vi "Send Time-delayed Transfer Sample.vi"(8 "error in (no error)":errorcluster, 9 "Milliseconds To Wait (1000)":i32=1000, 11 "cRIO-CO2 in":refnum<class "cRIO-CO2.lvclass">) -> (0 "error out":errorcluster, 3 "cRIO-CO2 out":refnum<class "cRIO-CO2.lvclass">)   [LabVIEW 2015, in "cRIO-Carbondioxide.lvlib" / "cRIO-CO2.lvlib" / "cRIO-CO2.lvclass"]
uses:
  cRIO-CO2.lvclass
  cRIO-CO2 Messages/Transfer Sample Msg/Transfer Sample Msg.lvclass
  <vilib>/ActorFramework/Time-Delayed Send Message/Time-Delay Override Options.ctl
  <vilib>/ActorFramework/Message/Message.lvclass
  cRIO-CO2.lvclass/cRIO-CO2.ctl
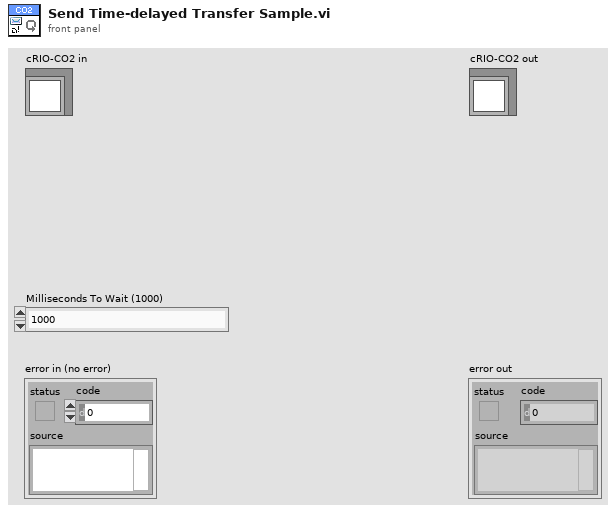
[diagram p1: front panel]
types:
  T1 = typedef "Time-Delay Override Options.ctl" = enum16{"Send next copy now", "Skip next scheduled copy", "Send next copy now and stop all further copies", "Stop all further copies"}
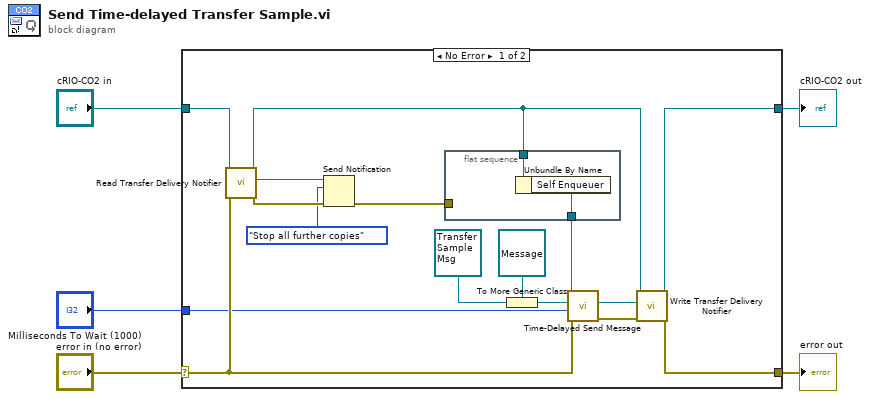
[diagram p0: block diagram]
diagram:
  n1 = case shown="No Error" "error in (no error)" {
    selector: "error in (no error)" -> [w16 w25]
    tunnel: [w17 w25] -> w4
    tunnel: [w18 w24] -> w2
    tunnel: "cRIO-CO2 in" -> [w15 w24]
    tunnel: "Milliseconds To Wait (1000)" -> [w10 _]
    frame No Error {
      n2 = call "Read Transfer Delivery Notifier.vi"("error in (no error)"=w16, "cRIO-CO2 in"=w15) -> ("error out"=w12:errorcluster, "Transfer Delivery Notifier"=w13:refnum<notifier>, "cRIO-CO2 out"=w14:refnum<class "cRIO-CO2.lvclass">)  [unwired: 7 in]
      n3 = Send Notification(notification=Time-Delay_Override_Options."Stop all further copies", notifier=w13, error in (no error)=w12) -> (error out=w6:errorcluster)  [unwired: 1 out]
      n4 = flat-sequence {
        tunnel: [w23] -> w21
        tunnel: w14 -> [w22]
        tunnel: w6 -> [_]
        frame #0 {
          n5 = Unbundle By Name(w22) -> ("Self Enqueuer"=w23:refnum<class "Message Enqueuer.lvclass">)
        }
      }
      n6 = To More Generic Class(target class=refnum<class "Message.lvclass"> refnum ("Message"), reference=refnum<class "Transfer Sample Msg.lvclass"> refnum ("Transfer Sample Msg.lvclass")) -> (generic class reference=w7:refnum<class "Message.lvclass">)
      n7 = call <vilib>:"Time-Delayed Send Message.vi"("error in (no error)"=w16, "Milliseconds To Wait"=w10, "Message"=w7, "Message Enqueuer"=w21) -> ("error out"=w20:errorcluster, "Delivery Notifier"=w19:refnum<notifier>)  [unwired: 6 in]
      n8 = call "Write Transfer Delivery Notifier.vi"("error in (no error)"=w20, "Transfer Delivery Notifier"=w19, "cRIO-CO2 in"=w14) -> ("error out"=w17:errorcluster, "cRIO-CO2 out"=w18:refnum<class "cRIO-CO2.lvclass">)  [unwired: 7 in]
    }
    frame Error {
    }
  }
  "error out" <- w4
  "cRIO-CO2 out" <- w2
